vi "Get RHS.vi"(8 "error in (no error)":errorcluster, 10 "Domain":refnum<class "NI_Domain.lvclass">, 11 "RHS in":refnum<class "NI_RHS.lvclass">) -> (0 "error out":errorcluster, 2 "RHS":variant, 3 "RHS out":refnum<class "NI_RHS.lvclass">)   [LabVIEW 2017, in "NI_PDE.lvlib" / "NI_RHS.lvclass"]
uses:
  <vilib>/gmath/pde.llb/RHSClass/NI_RHS.lvclass
  <vilib>/gmath/pde.llb/DomainClass/NI_Domain.lvclass
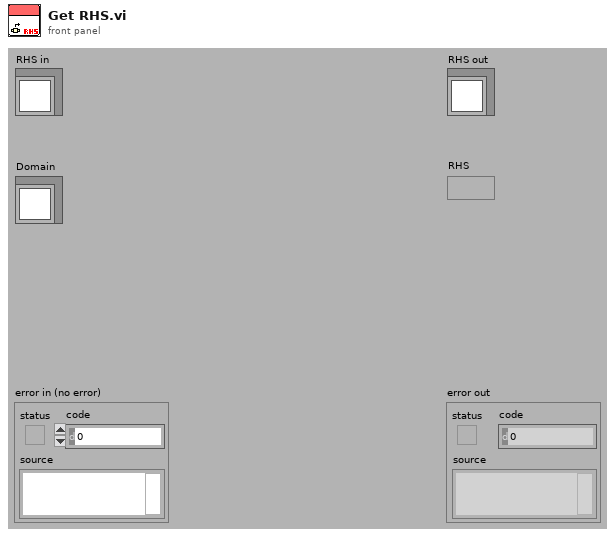
[diagram p1: front panel]
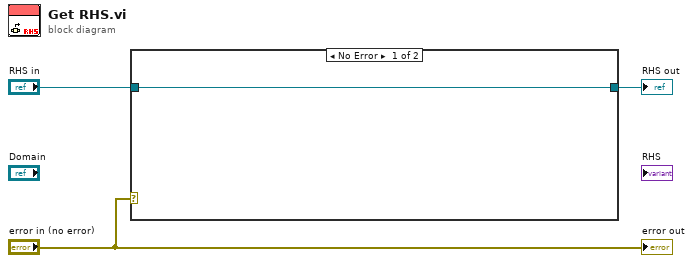
[diagram p0: block diagram]
diagram:
  n1 = case shown="No Error" "error in (no error)" {
    tunnel: "RHS in" -> [w4 w5]
    tunnel: [w4 w5] -> w2
    frame No Error {
    }
    frame Error {
    }
  }
  "RHS out" <- w2
  "error out" <- "error in (no error)"
